vi "Parse ERD Read Results.vi"(0 "Verify ERD Response?":bool=TRUE, 2 "Read ERD List":T2[](array[typedef]) {"ERD Number" format="%.0x"}, 5 "Raw Message":string, 7 "Converted Data":T3 {"CRC" format="%04x"; "Length" format="%02x"; "Command" format="%02x"; "Destination" format="%02x"; "Source" format="%02x"}, 11 "Error In":errorcluster) -> (4 "Pass/Fail?":bool, 8 "ERD Data Out":T1[](array[typedef]) {"ERD Number" format="%.0x"}, 15 "Error Out":errorcluster)   [LabVIEW 2023]
doc: "This VI takes the converted return data from the GEA2 Send and Receive and formats the Data based on the selections made in the Read ERD list. In addition, it also verifies the ERDs requested were returned."
uses:
  type defs/Data Out.ctl
  type defs/ERD Read Data In.ctl
  type defs/ERD Read Data Out.ctl
  library/GEA2_Toolkit.lvlib
panel:
  out "size(s)":i32
  out "String 2":string
  out "concatenated string":string
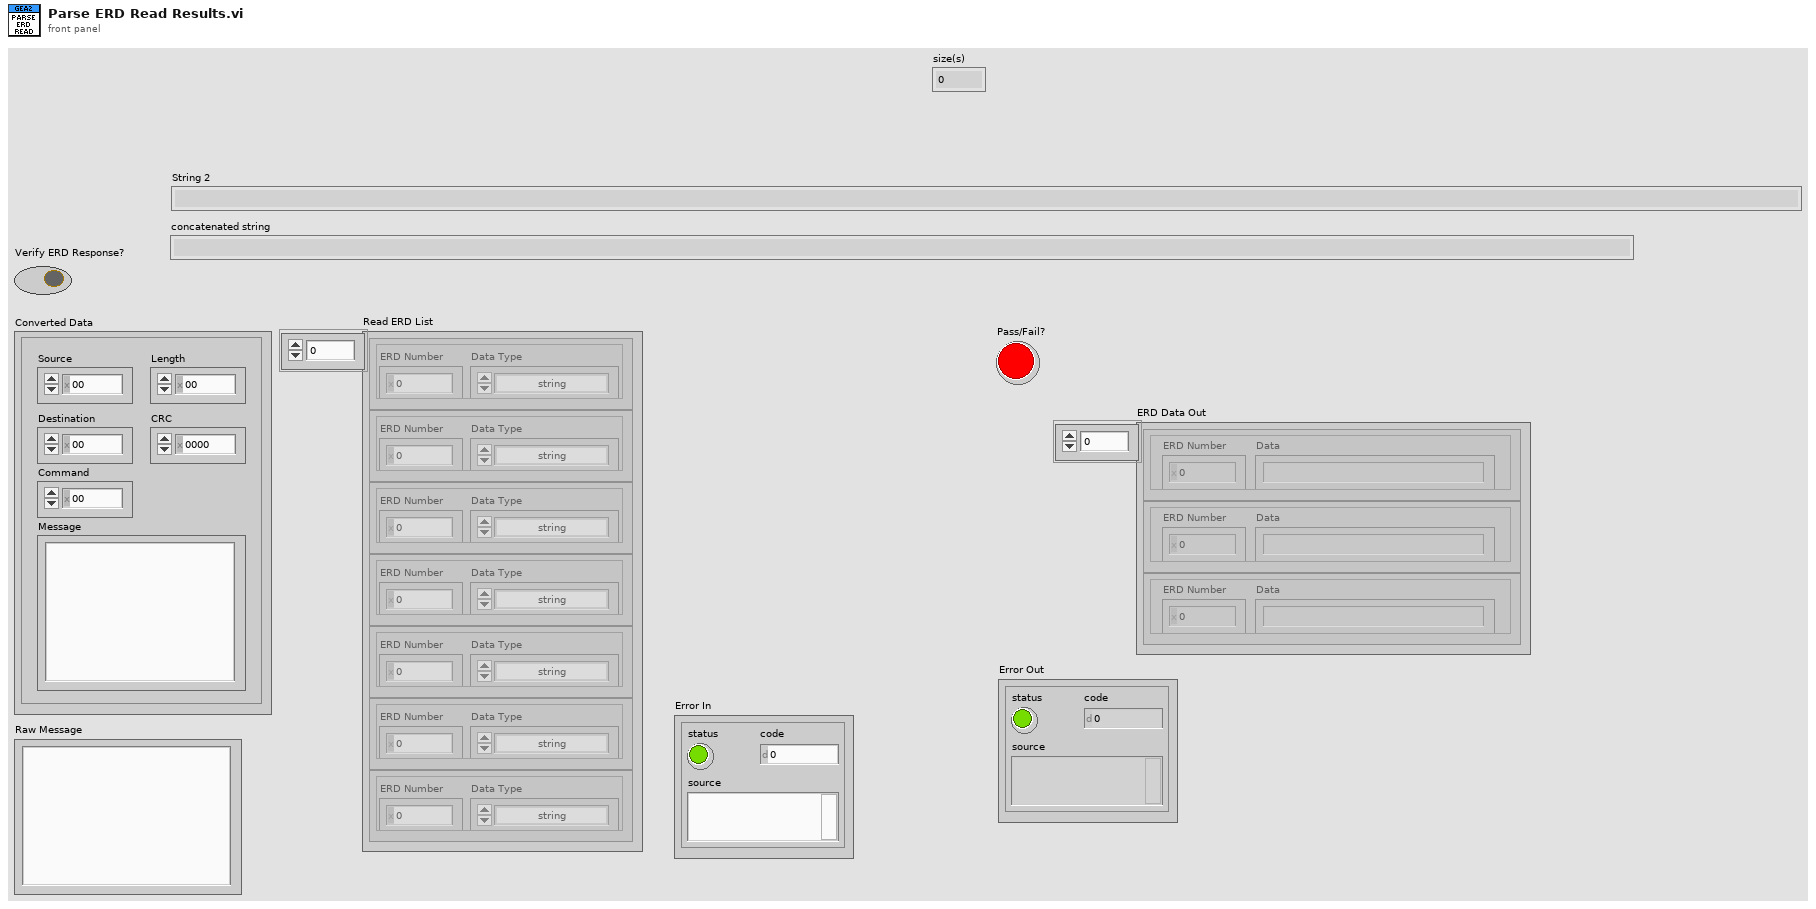
[diagram p1: front panel]
types:
  T1 = typedef "ERD Read Data Out.ctl" = cluster{"ERD Number":u16, "Data":string}
  T2 = typedef "ERD Read Data In.ctl" = cluster{"ERD Number":u16, "Data Type":enum16{"string", "boolean", "uint8_t", "uint16_t", "uint32_t", "uint64_t", "int8_t", "int16_t", "int32_t", "int64_t"}}
  T3 = typedef "GEA2_Toolkit.lvlib/Data Out.ctl" = cluster{"Source":u8, "Destination":u8, "Command":u8, "Length":u8, "CRC":u16, "Message":string}
  T4 = enum16{"string", "boolean", "uint8_t", "uint16_t", "uint32_t", "uint64_t", "int8_t", "int16_t", "int32_t", "int64_t"}
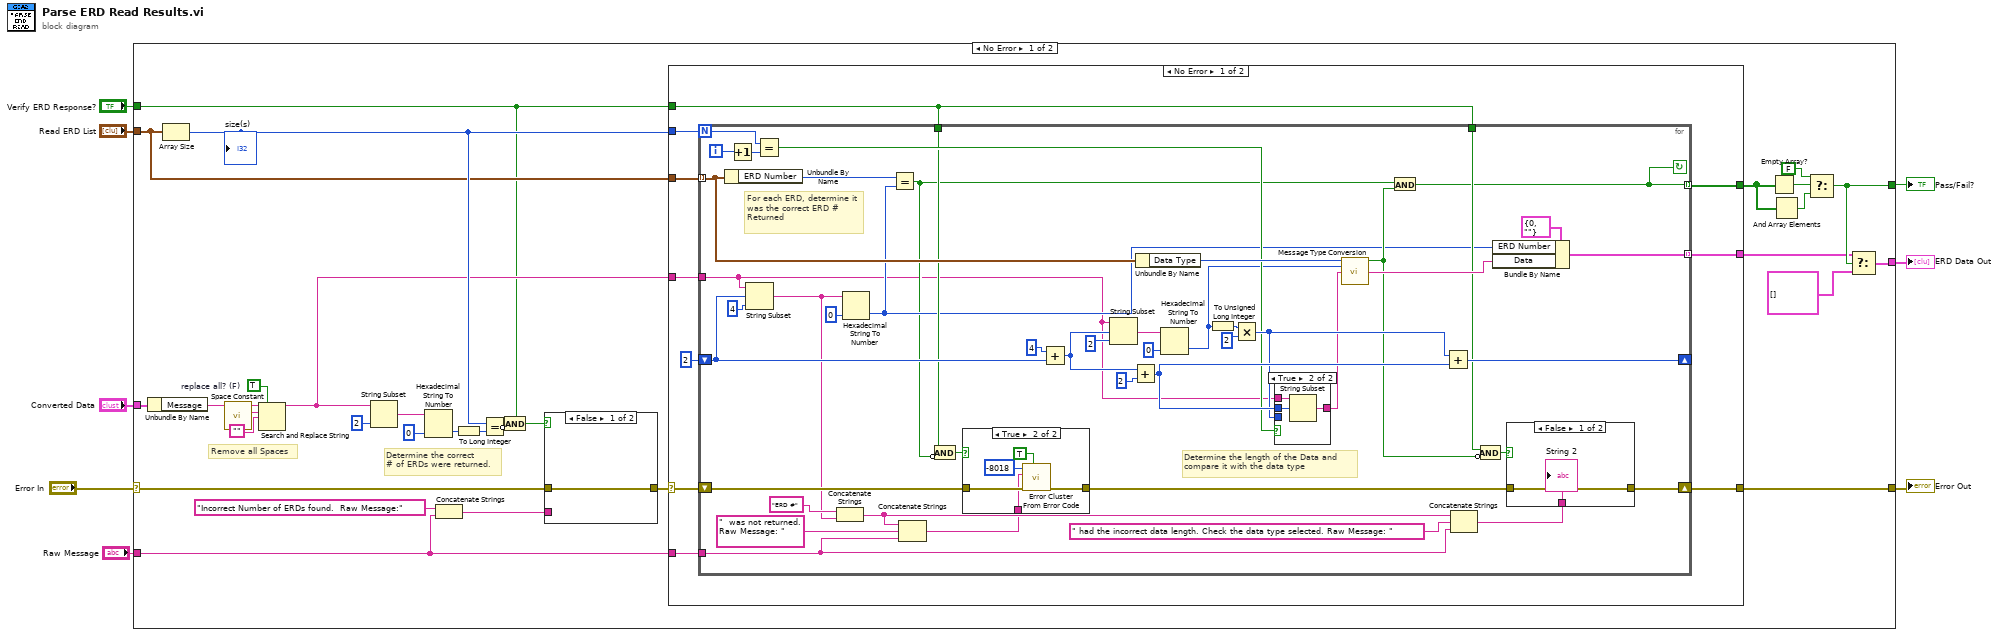
[diagram p0: block diagram]
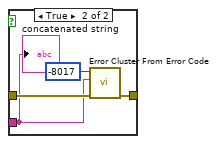
[diagram p2: hidden frame]
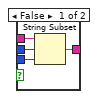
[diagram p3: hidden frame]
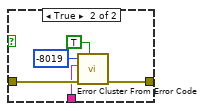
[diagram p5: hidden frame]
diagram:
  n1 = case shown="No Error" "Error In" {
    selector: "Error In" -> [w19 w121]
    tunnel: "Converted Data" -> [w38 _]
    tunnel: "Read ERD List" -> [w31 _]
    tunnel: [w27 _] -> w2
    tunnel: [w11 _] -> w1
    tunnel: [w20 w121] -> w5
    tunnel: "Raw Message" -> [w15 _]
    tunnel: "Verify ERD Response?" -> [w14 _]
    frame No Error {
      w21 = TRUE  # replace all? (F)
      # "Remove all Spaces"
      # "Determine the correct \n# of ERDs were returned."
      n2 = Unbundle By Name(w38) -> ("Message"=w23:string)
      n3 = Array Size(array=w31) -> (size(s)=w34:i32)
      "size(s)" <- w34
      n4 = call <vilib>:"Space Constant.vi"() -> ("String"=w25:string)
      n5 = Search and Replace String(replace all?=w21, input string=w23, search string=w25, replace string="") -> (result string=w22:string)  [unwired: 4 in, 3 out]
      n6 = String Subset(string=w22, length (rest)=2 ("length (rest)")) -> (substring=w36:string)  [unwired: 1 in]
      n7 = Hexadecimal String To Number(string=w36, default (0uL)=u8 0) -> (number=w32:u8)  [unwired: 1 in, 1 out]
      n8 = Concatenate Strings("Incorrect Number of ERDs found.  Raw Message:" ("string"), w15) -> (w17:string)
      n9 = To Long Integer(number=w32) -> (32bit integer=w33:i32)
      n10 = Equal?(x=w34, y=w33) -> (x = y?=w13:bool)
      n11 = Compound Arithmetic op=AND(w14, invert w13) -> (w12:bool)
      n12 = case shown="False" w12 {
        tunnel: [w39 w43] -> w16
        tunnel: w19 -> [w39 w41]
        tunnel: w17 -> [_ w40]
        frame False {
        }
        frame True {
          n13 = call <vilib>:"Error Cluster From Error Code.vi"("error in (no error)"=w41, "error message (\"\")"=w40, "error code (0)"=-8017) -> ("error out"=w43:errorcluster)  [unwired: 6 in]
          "concatenated string" <- w40
        }
      }
      n14 = case shown="No Error" w16 {
        selector: w16 -> [w49 w120]
        tunnel: w34 -> [w53 _]
        tunnel: [w44 _] -> w30
        tunnel: w22 -> [w52 _]
        tunnel: w31 -> [w51 _]
        tunnel: [w45 _] -> w9
        tunnel: [w50 w120] -> w20
        tunnel: w15 -> [w48 _]
        tunnel: w14 -> [w46 _]
        frame No Error {
          n15 = for {
            N: w53 -> [w70]
            tunnel: w52 -> [w54]
            shift-right: [w86] -> _
            shift-left: u32 2 -> [w87]
            tunnel: w51 -> [w90] mode=indexing
            tunnel: [w55] -> w45 mode=indexing
            tunnel: [w61] -> w44 mode=indexing
            shift-right: [w95] -> w50
            shift-left: w49 -> [w92]
            tunnel: w48 -> [w80]
            tunnel: w46 -> [w67]
            tunnel: w46 -> [w64]
            i -> [w94]
            stop <- w61 continue-if-true
            # "For each ERD, determine it was the correct ERD # Returned"
            # "Determine the length of the Data and\ncompare it with the data type"
            n16 = Unbundle By Name(w90) -> ("ERD Number"=w57:u16)
            n17 = Increment(x=w94) -> (x+1=w93:i32)
            n18 = String Subset(string=w54, offset (0)=w87, length (rest)=4 ("length (rest)")) -> (substring=w58:string)
            n19 = Equal?(x=w70, y=w93) -> (x = y?=w69:bool)
            n20 = Concatenate Strings("ERD #" ("string"), w58) -> (w83:string)
            n21 = Hexadecimal String To Number(string=w58, default (0uL)=u16 0) -> (number=w59:u16)  [unwired: 1 in, 1 out]
            n22 = Equal?(x=w57, y=w59) -> (x = y?=w56:bool)
            n23 = Concatenate Strings(w83, "  was not returned. Raw Message: " ("string"), w80) -> (w81:string)
            n24 = Compound Arithmetic op=AND(w67, invert w56) -> (w68:bool)
            n25 = case shown="True" w68 {
              tunnel: [w107 w112] -> w91
              tunnel: w92 -> [w107 w111]
              tunnel: w81 -> [_ w108]
              frame False {
              }
              frame True {
                n26 = call <vilib>:"Error Cluster From Error Code.vi"("show call chain? (False)"=TRUE, "error in (no error)"=w111, "error message (\"\")"=w108, "error code (0)"=-8018) -> ("error out"=w112:errorcluster)  [unwired: 5 in]
              }
            }
            n27 = Add(x=u32 4, y=w87) -> (x+y=w73:u32)
            n28 = String Subset(string=w54, offset (0)=w73, length (rest)=2 ("length (rest)")) -> (substring=w77:string)
            n29 = Add(x=w73, y=u32 2) -> (x+y=w72:u32)
            n30 = Unbundle By Name(w90) -> ("Data Type"=w89:T4)
            n31 = Hexadecimal String To Number(string=w77, default (0uL)=u8 0 ("default (0 U32)")) -> (number=w62:u8)  [unwired: 1 in, 1 out]
            n32 = To Unsigned Long Integer(number=w62) -> (unsigned 32bit integer=w63:u32)
            n33 = Multiply(x=w63, y=u32 2) -> (x*y=w71:u32)
            n34 = case shown="True" w69 {
              tunnel: w54 -> [w103 w106]
              tunnel: w72 -> [w101 w105]
              tunnel: [w102 w104] -> w60
              tunnel: w71 -> [w100 _]
              frame False {
                n35 = String Subset(string=w103, offset (0)=w101, length (rest)=w100) -> (substring=w102:string)
              }
              frame True {
                n36 = String Subset(string=w106, offset (0)=w105) -> (substring=w104:string)  [unwired: 1 in]
              }
            }
            n37 = call "Message Type Conversion.vi"("Data Type"=w89, "Data Length"=w62, "Message In"=w60) -> ("Pass/Fail?"=w66:bool, "Message Out"=w96:string)  [unwired: 11 in]
            n38 = And(x=w56, y=w66) -> (x .and. y?=w61:bool)
            n39 = Add(x=w71, y=w72) -> (x+y=w86:u32)
            n40 = Concatenate Strings(w83, " had the incorrect data length. Check the data type selected. Raw Message: " ("string"), w80) -> (w79:string)
            n41 = Compound Arithmetic op=AND(w64, invert w66) -> (w65:bool)
            n42 = Bundle By Name(cluster=T1 {"ERD Number"=0, "Data"=""} ("ERD Output"), "ERD Number"=w59, "Data"=w96) -> (w55:T1)
            n43 = case shown="False" w65 {
              tunnel: [w114 w119] -> w95
              tunnel: w91 -> [w114 w118]
              tunnel: w79 -> [w113 w115]
              frame False {
                "String 2" <- w113
              }
              frame True {
                n44 = call <vilib>:"Error Cluster From Error Code.vi"("show call chain? (False)"=TRUE, "error in (no error)"=w118, "error message (\"\")"=w115, "error code (0)"=-8019) -> ("error out"=w119:errorcluster)  [unwired: 5 in]
              }
            }
          }
        }
        frame Error {
        }
      }
      n45 = Empty Array?(array=w30) -> (empty?=w29:bool)
      n46 = And Array Elements(Boolean array=w30) -> (logical AND=w10:bool)
      n47 = Select(t=FALSE, s=w29, f=w10) -> (s? t:f=w27:bool)
      n48 = Select(t=w9, s=w27, f=T1[] []) -> (s? t:f=w11:T1[])
    }
    frame Error {
    }
  }
  "Pass/Fail?" <- w2
  "ERD Data Out" <- w1
  "Error Out" <- w5
